vi "Test_read_version_app.vi"() -> ()   [LabVIEW 2018]
uses:
  <vilib>/Utility/config.llb/Read Key (String).vi
  <vilib>/Utility/config.llb/NI_LVConfig.lvlib
panel:
  out "ver":string
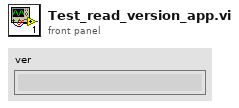
[diagram p1: front panel]
types:
  T1 = typedef "NI_LVConfig.lvlib/Config Data RefNum.ctl" = refnum<k1>
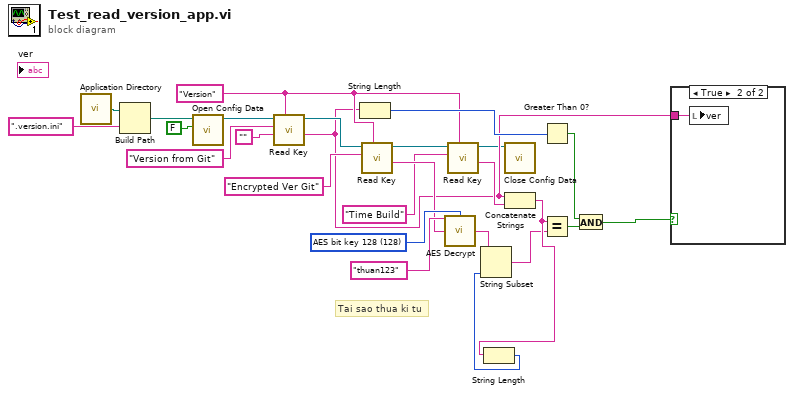
[diagram p0: block diagram]
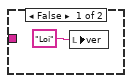
[diagram p2: hidden frame]
diagram:
  w16 = u16 128 items=["AES bit key 128"=128, "AES bit key 192"=192, "AES bit key 256"=256] ("BitKeyType(256)")
  w9 = "Version" ("key")
  # "Tai sao thua ki tu"
  n1 = call <vilib>:"Application Directory.vi"() -> ("Application Directory"=w26:path)
  n2 = Build Path(base path=w26, name or relative path=".version.ini") -> (appended path=w24:path)
  n3 = call <vilib>:"Open Config Data.vi"("create file if necessary (T)"=FALSE, "configuration file path"=w24) -> ("refnum"=w21:T1)  [unwired: 1 in, 8 out]
  n4 = call-poly <vilib>:"Read Key.vi"("section"=w9, "default value"="", "key"="Version from Git", "refnum"=w21) -> ("value"=w7:string, "refnum out"=w18:T1)  [unwired: 4 in, 2 out]
  n5 = String Length(string=w7) -> (length=w19:i32)
  n6 = call-poly <vilib>:"Read Key.vi"("section"=w9, "key"="Encrypted Ver Git", "refnum"=w18) -> ("value"=w14:string, "refnum out"=w6:T1)  [unwired: 5 in, 2 out]
  n7 = call "AES Decrypt.vi"("Password.In"="thuan123", "BitKeyType(256)"=w16, "EncryptedText.In"=w14) -> ("DecryptedText.Out"=w4:string)  [unwired: 11 in, 1 out]
  n8 = call-poly <vilib>:"Read Key.vi"("section"=w9, "key"="Time Build", "refnum"=w6) -> ("value"=w8:string, "refnum out"=w5:T1)  [unwired: 5 in, 2 out]
  n9 = call <vilib>:"Close Config Data.vi"("refnum"=w5) -> ()  [unwired: 2 in, 9 out]
  n10 = Concatenate Strings(w7, w8) -> (w3:string)
  n11 = String Length(string=w3) -> (length=w2:i32)
  n12 = String Subset(string=w4, length (rest)=w2) -> (substring=w1:string)  [unwired: 1 in]
  n13 = Greater Than 0?(x=w19) -> (x > 0?=w11:bool)
  n14 = Equal?(x=w3, y=w1) -> (x = y?=w12:bool)
  n15 = And(x=w11, y=w12) -> (x .and. y?=w13:bool)
  n16 = case shown="True" w13 {
    tunnel: w7 -> [_ w28]
    frame False {
      n17 = local write "ver"("Loi" ("ver")) -> ()
    }
    frame True {
      n18 = local write "ver"(w28) -> ()
    }
  }
